vi "Init Transport.vi"() -> (2 "Transport":refnum<class "Transport.lvclass">)   [LabVIEW 2025, in "jettl.lvlib" / "Transport.lvlib" / "Event.lvlib"]
uses:
  Event.lvlib
  Transport/Transport.lvclass
  Event Transport/Event Transport.lvclass
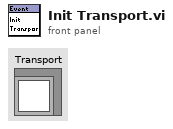
[diagram p1: front panel]
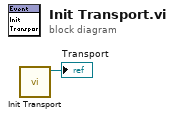
[diagram p0: block diagram]
diagram:
  n1 = call "Init Transport.vi"() -> ("Event Transport out"=→"Transport":refnum<class "Event Transport.lvclass">)  [unwired: 11 in]
